vi "Read.vi"(10 "Address":u16 format="%04x", 11 "EEPROM in":refnum<class "EEPROM.lvclass">) -> (3 "Data":u8 format="%02x")   [LabVIEW 2021, in "EEPROM.lvclass"]
uses:
  EEPROM.lvclass
  EEPROM.lvclass/EEPROM.ctl
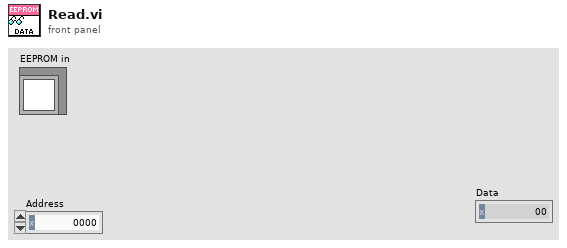
[diagram p1: front panel]
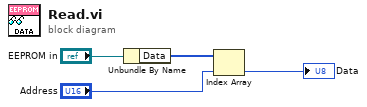
[diagram p0: block diagram]
diagram:
  n1 = Unbundle By Name("EEPROM in") -> ("Data"=w2:u8[])
  n2 = Index Array(array=w2, index="Address") -> (element=→"Data":u8)
